vi "StartProcess.vi"(7 "Process":T1, 8 "error in (no error)":errorcluster, 10 "externalProcess?":bool, 11 "viToLaunchInfos":T2={"File Path Control"=path "", "Timeout"=10.0, "viInitString"="", "State"=enum."Hidden"}) -> (0 "error out":errorcluster)   [LabVIEW 2011]
uses:
  050 - CONFIG/20 - ExternalProcesses/paramsExternalProcesses.ctl
  EnumProcess.ctl
  EnumFgvReferenceProcess.ctl
  030 - EVENTS/EnumFgvEventCommand.ctl
  090 - ERRORS/Ctrls/EnumErrors.ctl
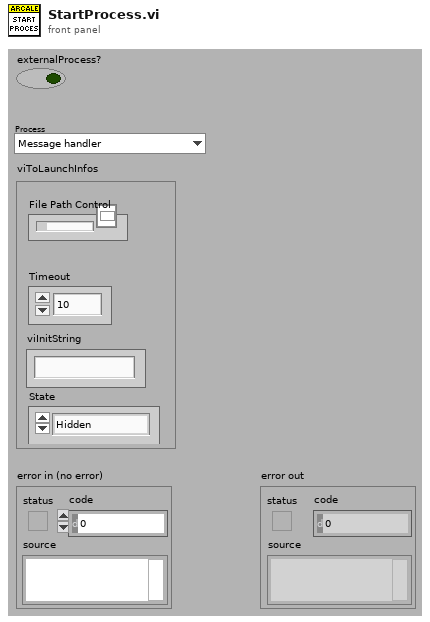
[diagram p1: front panel]
types:
  T1 = typedef "EnumProcess.ctl" = enum16{"Message handler", "Template"}
  T2 = typedef "paramsExternalProcesses.ctl" = cluster{"File Path Control":path, "Timeout":dbl, "viInitString":string, "State":enum32{"Invalid", "Standard", "Closed", "Hidden", "Minimized", "Maximized"}}
  T3 = typedef "EnumFgvReferenceProcess.ctl" = enum16{"Init", "Get", "Add Reference", "Close References"}
  T4 = typedef "EnumFgvEventCommand.ctl" = enum16{"Setup", "Cleanup", "Get"}
  T5 = typedef "EnumErrors.ctl" = enum16{"VI non trouvé !", "Clé non trouvée", "Timeout", "Le VI tourne déjà", "Erreur de séparateur décimal", "Référence non trouvée"}
  T6 = enum32{"Invalid", "Standard", "Closed", "Hidden", "Minimized", "Maximized"}
  T7 = typedef "FromProcessesEventType.ctl" = enum16{"Started", "Autotest", "Ended"}
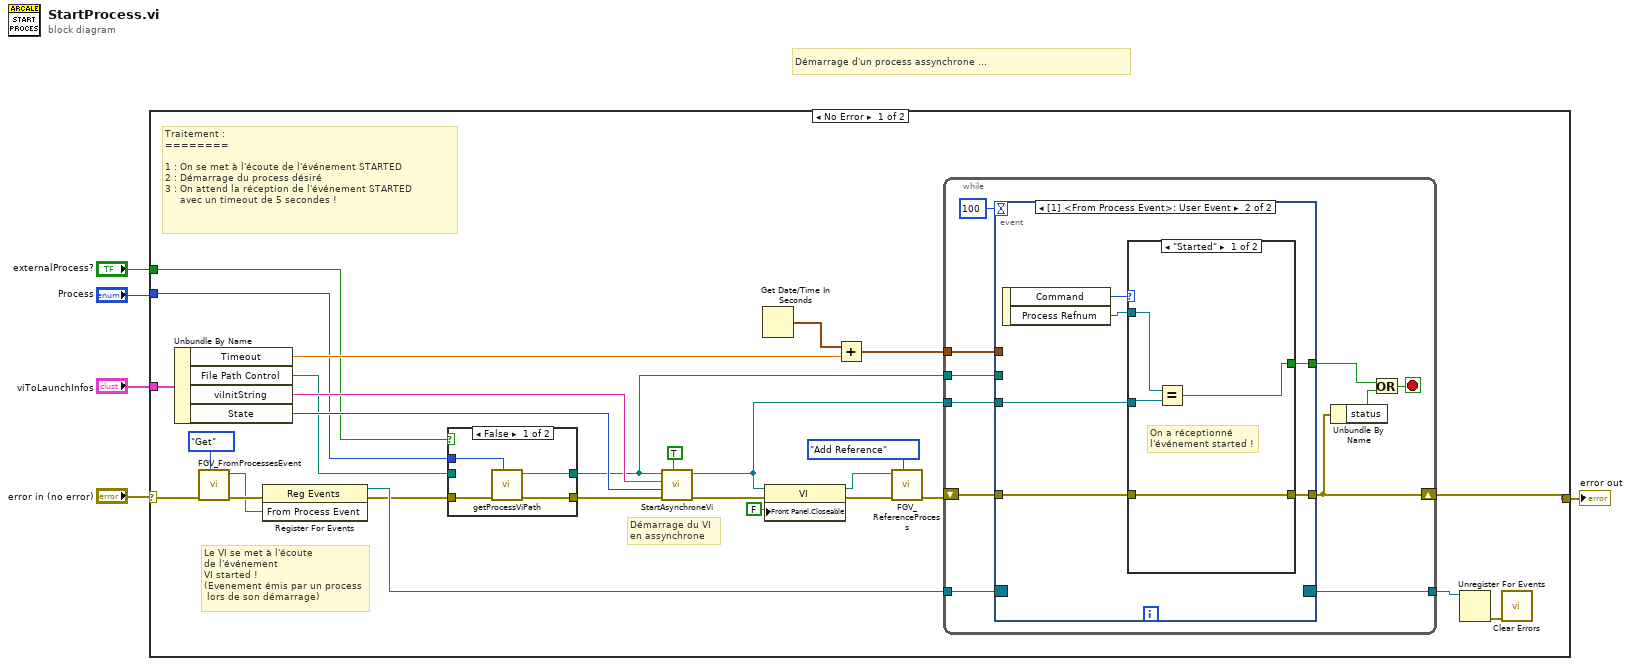
[diagram p0: block diagram]
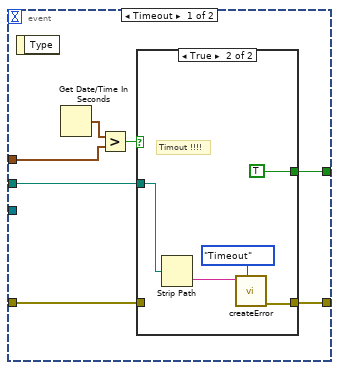
[diagram p3: hidden frame]
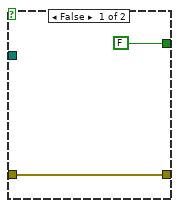
[diagram p4: hidden frame]
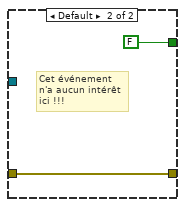
[diagram p5: hidden frame]
diagram:
  # "Démarrage d'un process assynchrone ..."
  n1 = case shown="No Error" "error in (no error)" {
    selector: "error in (no error)" -> [w27 w77]
    tunnel: [w20 w77] -> w4
    tunnel: "viToLaunchInfos" -> [w16 _]
    tunnel: "Process" -> [w11 _]
    tunnel: "externalProcess?" -> [w12 _]
    frame No Error {
      # "Traitement :\n========\n\n1 : On se met à l'écoute de l'événement STARTED\n2 : Démarrage du process désiré\n3 : On attend la réception de l'événement STARTED\n     avec un timeout de 5 secondes !"
      # "Le VI se met à l'écoute\nde l'événement \nVI started !\n(Evenement émis par un process\n lors de son démarrage)"
      # "Démarrage du VI \nen assynchrone"
      n2 = Unbundle By Name(w16) -> ("Timeout"=w15:dbl, "File Path Control"=w10:path, "viInitString"=w14:string, "State"=w13:T6)
      n3 = call "FGV_FromProcessesEvent.vi"("Command"=EnumFgvEventCommand."Get", "error in (no error)"=w27) -> ("error out"=w32:errorcluster, "From Process Event"=w21:refnum<user-event>)  [unwired: 8 in]
      n4 = register-events(error in=w32, w21) -> (reference out=w19:refnum<event-registration>, error out=w8:errorcluster)  [unwired: 1 in]
      n5 = case shown="False" w12 {
        tunnel: w11 -> [w37 _]
        tunnel: [w36 w39] -> w9
        tunnel: w10 -> [_ w39]
        tunnel: w8 -> [w35 w38]
        tunnel: [w34 w38] -> w7
        frame False {
          n6 = call "getProcessViPath.vi"("Enum Screen"=w37, "error in (no error)"=w35) -> ("error out"=w34:errorcluster, "Path"=w36:path)  [unwired: 8 in]
        }
        frame True {
        }
      }
      n7 = call "StartAsynchroneVi.vi"("Open Front Panel ?"=TRUE, "error in"=w7, "State"=w13, "viInitString"=w14, "viPathToStart"=w9) -> ("error out"=w24:errorcluster, "vi reference"=w6:refnum<vi>)  [unwired: 5 in]
      n8 = Get Date/Time In Seconds() -> (seconds since 1Jan1904=w31:timestamp)
      n9 = property class="VI"(reference=w6, error in=w24, "Front Panel.Closeable"=FALSE ("Front Panel Window:Closeable")) -> (reference out=w18:refnum<vi>, error out=w23:errorcluster)
      n10 = Add(x=w31, y=w15) -> (x+y=w30:timestamp)
      n11 = call "FGV_ReferenceProcess.vi"("Commande"=EnumFgvReferenceProcess."Add Reference", "error in (no error)"=w23, "vi reference to add"=w18) -> ("error out"=w25:errorcluster)  [unwired: 7 in, 1 out]
      n12 = while {
        tunnel: w19 -> [w50]
        shift-right: [w46] -> w20
        shift-left: w25 -> [w42]
        tunnel: w30 -> [w49]
        tunnel: [w48] -> w29
        tunnel: w9 -> [w41]
        tunnel: w6 -> [w40]
        stop <- w43 stop-if-true
        n13 = event shown="[1] <From Process Event>: User Event" {
          selector: w50 -> [_ _]
          dyn-events: [_ _] -> w48
          timeout: 100 -> [_ _]
          tunnel: w42 -> [w55 w68]
          tunnel: [w53 w67] -> w46
          tunnel: w49 -> [w56 _]
          tunnel: [w52 w69] -> w44
          tunnel: w41 -> [w51 _]
          tunnel: w40 -> [_ w66]
          event Timeout {
            n14 = event-data() -> ()  [unwired: 1 in, 1 out]
            n15 = Get Date/Time In Seconds() -> (seconds since 1Jan1904=w57:timestamp)
            n16 = Greater?(x=w57, y=w56) -> (0:w54:bool)
            n17 = case shown="True" w54 {
              tunnel: w55 -> [w59 _]
              tunnel: [w59 w63] -> w53
              tunnel: [FALSE TRUE] -> w52
              tunnel: w51 -> [_ w60]
              frame False {
              }
              frame True {
                # "Timout !!!!"
                n18 = Strip Path(path=w60) -> (name=w61:string)  [unwired: 1 out]
                n19 = call "createError.vi"("ErrorCode"=EnumErrors."Timeout", "message"=w61) -> ("error out"=w63:errorcluster)  [unwired: 9 in]
              }
            }
          }
          event User Event {
            n20 = event-data() -> ("Command"=w70:T7, "Process Refnum"=w65:refnum<vi>)  [unwired: 1 in]
            n21 = case shown="\"Started\"" w70 {
              tunnel: [w71 FALSE] -> w69
              tunnel: w68 -> [w74 w75]
              tunnel: [w74 w75] -> w67
              tunnel: w66 -> [w73 _]
              tunnel: w65 -> [w72 _]
              frame "Started" {
                # "On a réceptionné \nl'événement started !"
                n22 = Equal?(x=w72, y=w73) -> (x = y?=w71:bool)
              }
              frame Default {
                # "Cet événement \nn'a aucun intérêt\nici !!!"
              }
            }
          }
        }
        n23 = Unbundle By Name(w46) -> ("status"=w45:bool)
        n24 = Or(x=w44, y=w45) -> (x .or. y?=w43:bool)
      }
      n25 = Unregister For Events(event registration refnum=w29) -> (error out=w28:errorcluster)  [unwired: 1 in]
      n26 = call <vilib>:"Clear Errors.vi"("error in (no error)"=w28) -> ()  [unwired: 6 in, 1 out]
    }
    frame Error {
    }
  }
  "error out" <- w4
